vi "Write Analogue.vi"(8 "error in (no error)":errorcluster, 10 "Output":bool, 11 "Keysight 5700C in":refnum<class "Keysight 5700C.lvclass">) -> (0 "error out":errorcluster, 3 "Keysight 5700C out":refnum<class "Keysight 5700C.lvclass">)   [LabVIEW 2021, in "Concrete.lvlib" / "Keysight 5700C.lvclass"]
uses:
  Keysight 5700C.lvclass
  Keysight 5700C.lvclass/Keysight 5700C.ctl
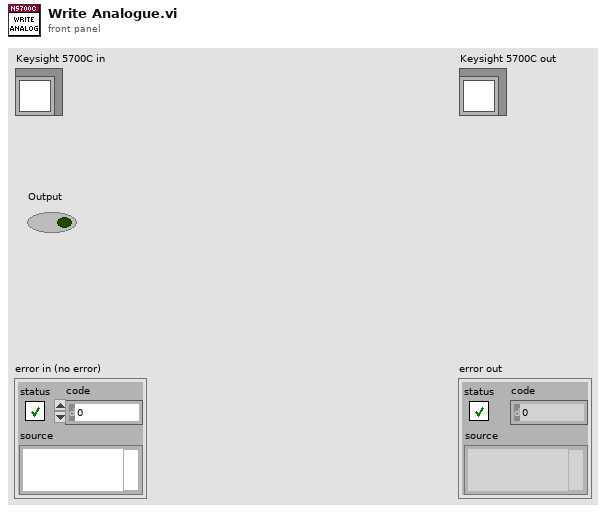
[diagram p1: front panel]
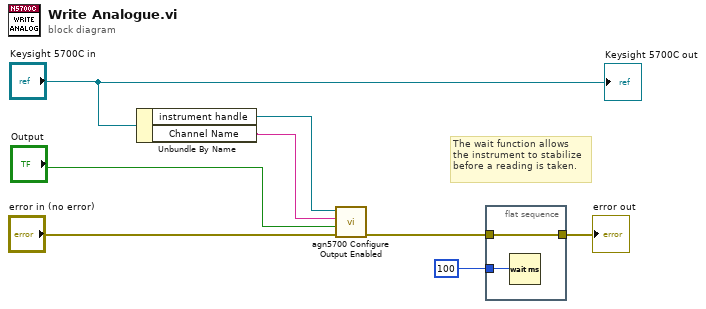
[diagram p0: block diagram]
diagram:
  # "The wait function allows \nthe instrument to stabilize\nbefore a reading is taken."
  n1 = Unbundle By Name("Keysight 5700C in") -> ("instrument handle"=w6:refnum<k15>, "Channel Name"=w5:string)
  n2 = call <instrlib>:"agn5700 Configure Output Enabled.vi"("error in (no error)"="error in (no error)", "enabled (True)"="Output", "channel name (\"\")"=w5, "instrument handle"=w6) -> ("error out"=w3:errorcluster)  [unwired: 7 out]
  n3 = flat-sequence {
    tunnel: [w10] -> w2
    tunnel: w3 -> [w10]
    tunnel: u32 100 ("milliseconds to wait") -> [w9]
    frame #0 {
      n4 = Wait (ms)(milliseconds to wait=w9) -> ()  [unwired: 1 out]
    }
  }
  "error out" <- w2
  "Keysight 5700C out" <- "Keysight 5700C in"
